vi "ncs_v4.vi"() -> ()   [LabVIEW 2016]
uses:
  <instrlib>/niUSRP/niUSRP Timestamp.ctl
  <vilib>/Analysis/3filter.llb/Filter Passband Type.ctl
  <instrlib>/niUSRP/niUSRP Write Tx Data (2D CDB).vi
  <instrlib>/niUSRP/niUSRP Fetch Rx Data (2D CDB).vi
  <vilib>/Analysis/baseanly.llb/IIR Cascade Filter (DBL).vi
  <vilib>/Analysis/NI_AALBase.lvlib
panel:
  in  "File Name":string="freq2G_1e"
  in  "Path":path=path "D:/Research/SummerFall17Spring18/CnC/NCS/Respiratory/Hexoskin/Data/3"
  out "NCS heartbeat":dbl[](graph)
  in  "Order":dbl=20.0 format="%#_13g"
  in  "High-Cutoff":dbl=8.0 format="%#_13g"
  in  "Low-Cutoff":dbl=0.5 format="%#_13g"
  out "size(s)":i32
  out "Coerced Rx IQ Rate":dbl
  in  "Sampling Rate":i32=500
  out "Gain":dbl=-15.0
  out "Bandwidth":dbl=56000000.0
  out "Coerced Carrier Freq":dbl=2000000000.0 format="%#.17g"
  out "Coerced Tx IQ rate":dbl=1000000.0
  out "error IO":errorcluster={"status"=FALSE, "code"=-1074118647, "source"=""}
  in  "Rx #Samples":i32=20000
  in  "Tab Control 2":enum32{"NI-294x/295x", "NI-2900/2901"}(tab)=enum."NI-2900/2901"
  in  "Rx carrier frequency [Hz]":dbl=2000000000.0 format="%#_6p"
  in  "Tx carrier frequency [Hz]":dbl=1000000000.0 format="%#_6p"
  in  "Start Trigger Time":T1={"whole seconds"=1, "fractional seconds"=0.0}
  in  "Tab Control":T2(tab)
  out "NCS tag Amp":dbl[](graph)=[0.011967714738528729, 0.012021355192189592, 0.012015275039596582, 0.011969166030167903, 0.011958890166168242, 0.012007893820858737, 0.012022893722444085, 0.011978222225113794, 0.011969989939463181, 0.012003099640895068]
  out "NCS tag Phase":dbl[](graph)=[0.011967714738528729, 0.012021355192189592, 0.012015275039596582, 0.011969166030167903, 0.011958890166168242, 0.012007893820858737, 0.012022893722444085, 0.011978222225113794, 0.011969989939463181, 0.012003099640895068]
  out "Tag Amp":dbl[](graph)
  out "Tag Phase":dbl[](graph)
  out "Tx Waveform Graph":waveform(dbl)[](graph)
  in  "Stop":bool
  in  "Tone Amplitude":dbl=0.707 step=0.05 format="%#.6g"
  in  "Tone Frequency":dbl=5000.0 format="%#_6p"
  in  "Tx Waveform Size":dbl=2000.0
  in  "Device Name":refnum<k15>="MyB210"
  in  "Tx Gain":dbl=28.0 format="%#_6f"
  in  "Tx IQ Rate":dbl=1000000.0 format="%#_6p"
  in  "Rx Gain":dbl=32.0 format="%#_6f"
  in  "Rx IQ Rate":dbl=500000.0 format="%#_6p"
  # "Note that on the NI-2900 and NI-2901, both Rx channels share an LO and both Tx channels share an LO. However, on the NI-294x/295x devices, Rx and Tx of channel 0 share an LO and Rx and Tx of channel 1 share an LO."
  # "Rx Settings"
  # "Tx Settings"
  # "Channel 0"
  # "Heartbeat Filter"
  # "This Tx graph should always have end and start tied up since this is being sent in a loop continuously. Otherwise phase jumps will be noticed."
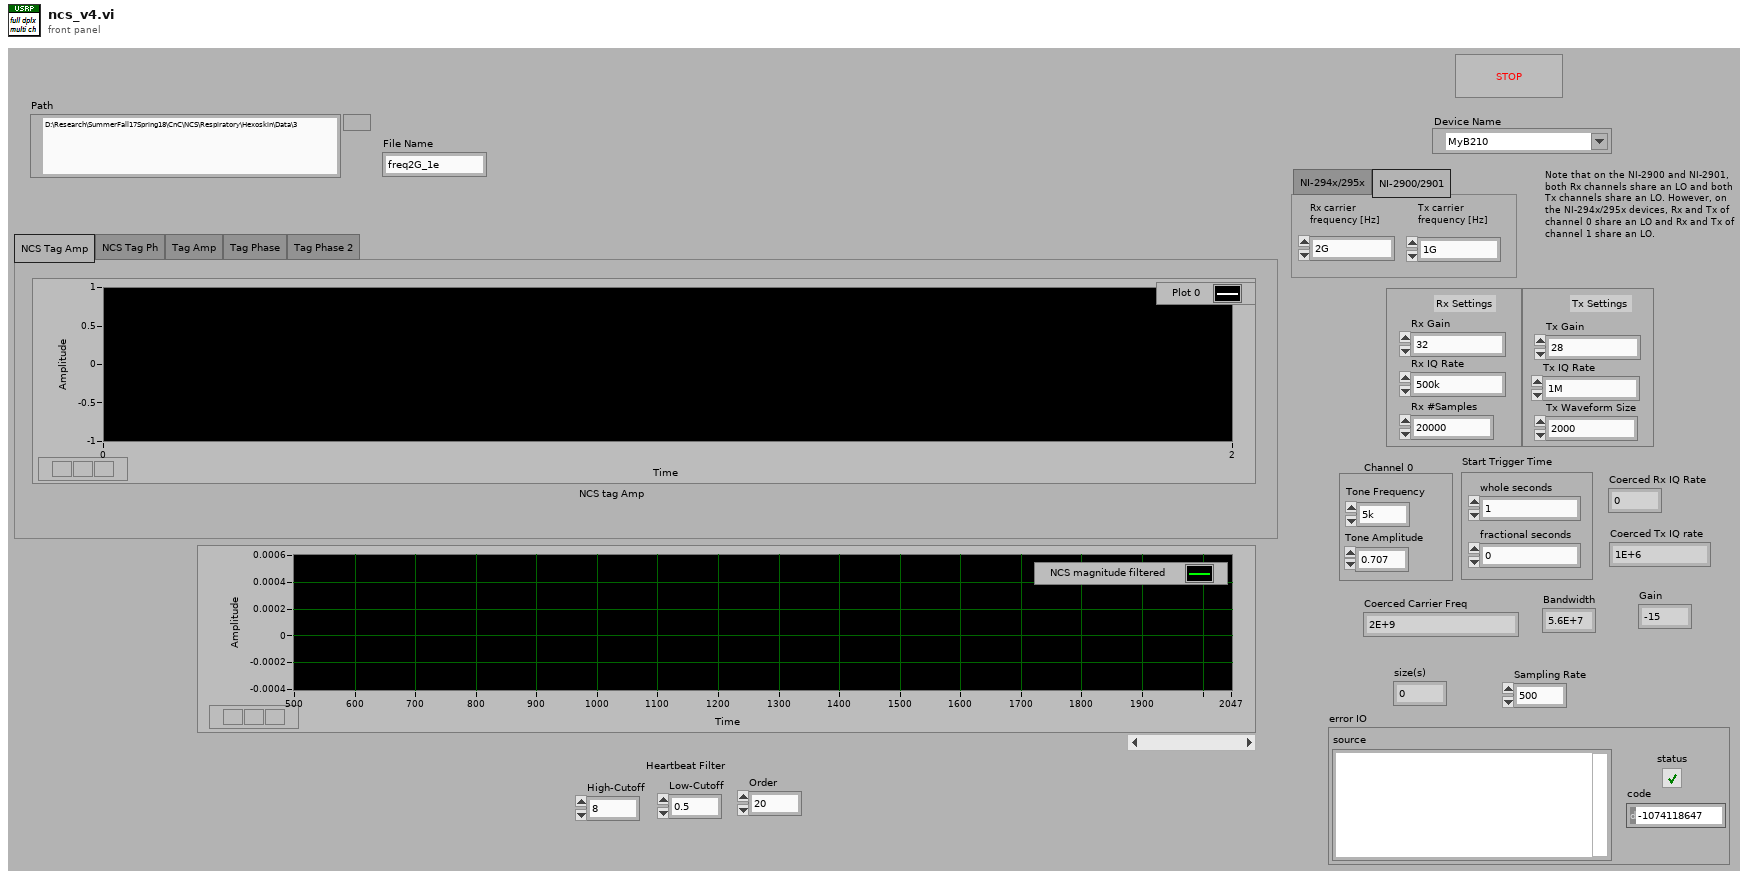
[diagram p1: front panel]
types:
  T1 = typedef "niUSRP Timestamp.ctl" = cluster{"whole seconds":u64, "fractional seconds":dbl}
  T2 = enum32{"NCS Tag Amp", "NCS Tag Ph", "Tag Amp", "Tag Phase", "Tag Phase 2"}
  T3 = typedef "NI_AALBase.lvlib/Filter Passband Type.ctl" = enum32{"Lowpass", "Highpass", "Bandpass", "Bandstop"}
  T4 = cluster{"filter structure":enum32{"IIR 2nd Order", "IIR 4th Order"}, "Reverse Coefficients":dbl[], "Forward Coefficients":dbl[]}
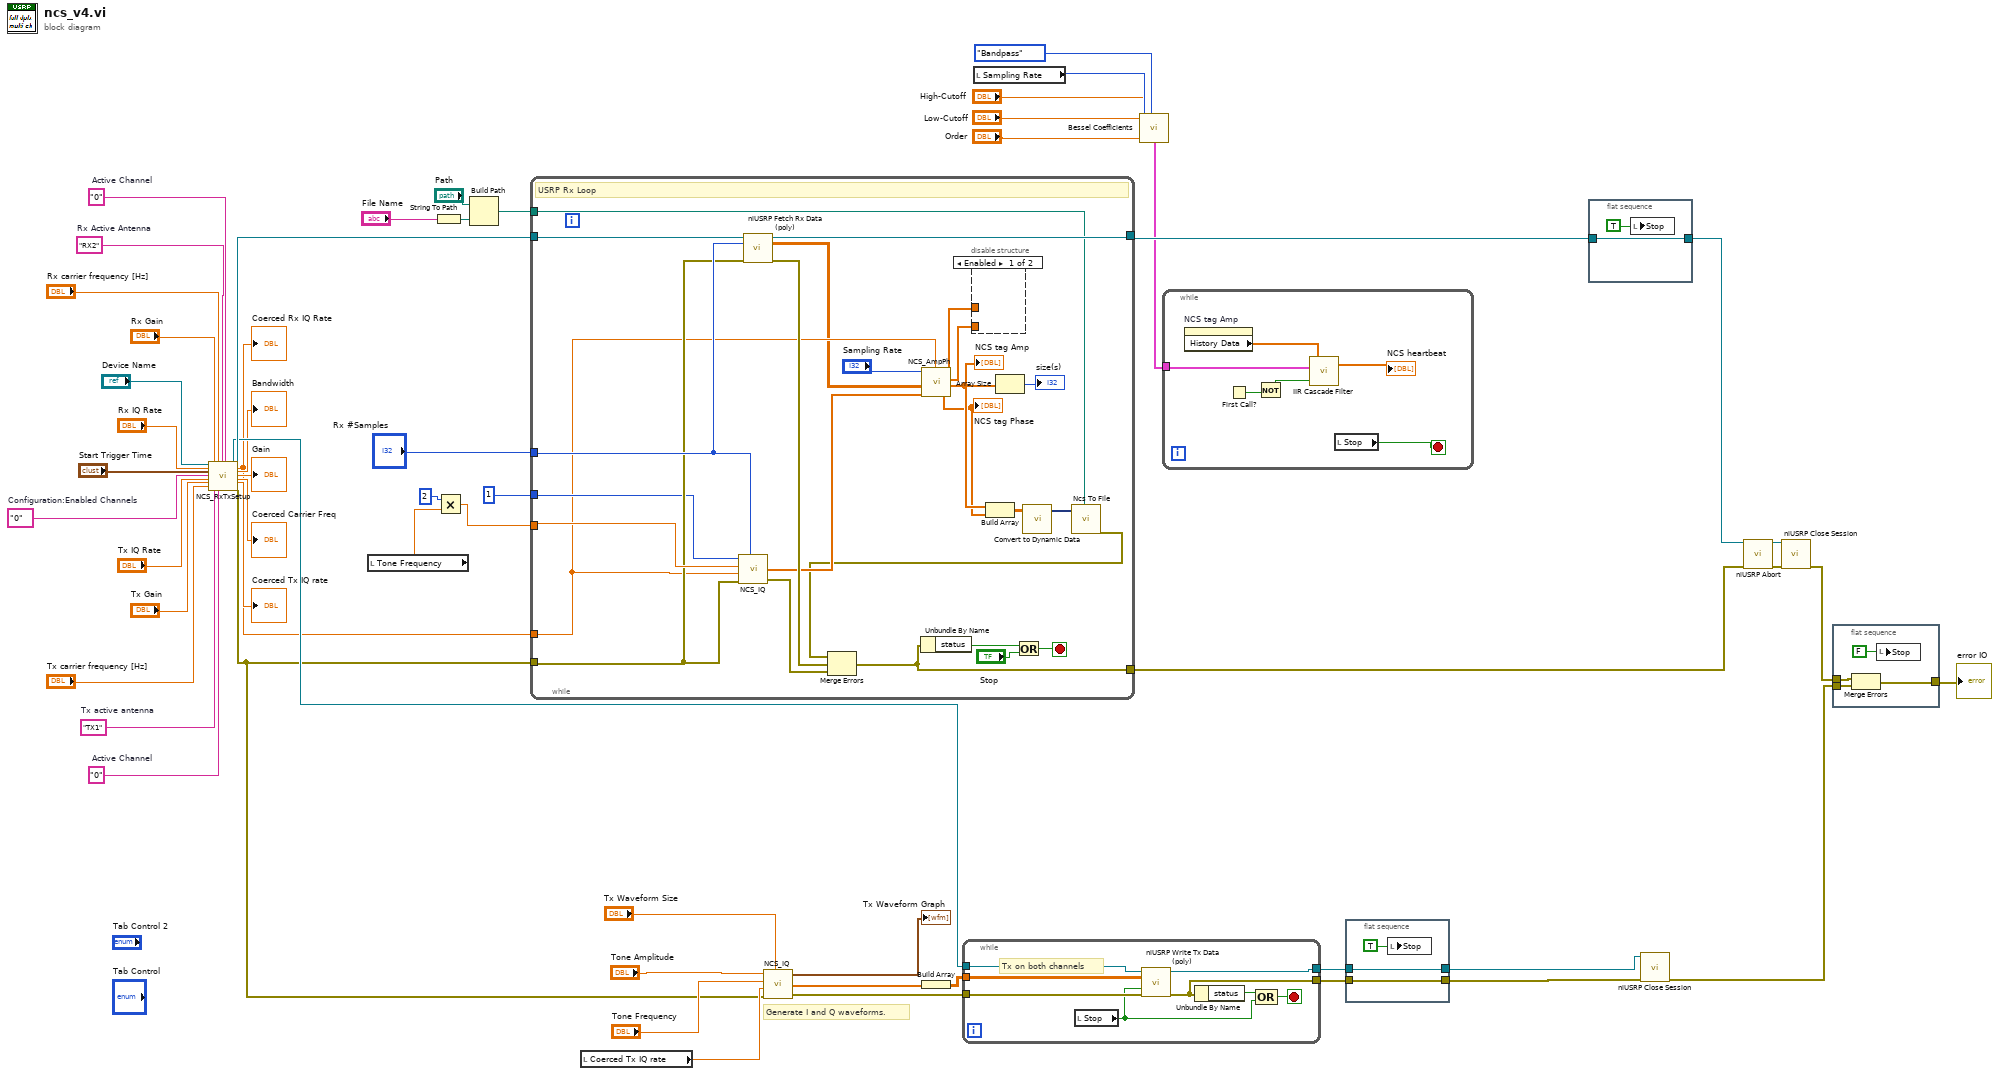
[diagram p0: block diagram]
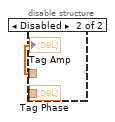
[diagram p2: hidden frame]
diagram:
  w12 = "0"  # Active Channel
  w13 = "0"  # Active Channel
  w48 = "RX2"  # Rx Active Antenna
  w44 = "TX1"  # Tx active antenna
  w30 = "0"  # Configuration:Enabled Channels
  # "Generate I and Q waveforms."
  n1 = call "NCS_RxTxSetup.vi"("IVI Refnum in"="Device Name", "Rx IQ Rate"="Rx IQ Rate", "Start Trigger Time"="Start Trigger Time", "Configuration:Enabled Channels"=w30, "Tx IQ Rate"="Tx IQ Rate", "Tx Gain"="Tx Gain", "Tx carrier frequency [Hz]"="Tx carrier frequency [Hz]", "Rx Gain"="Rx Gain", "Tx active antenna"=w44, "Rx carrier frequency [Hz]"="Rx carrier frequency [Hz]", "Active Channel"=w12, "Rx Active Antenna"=w48, "Active Channel 2"=w13) -> ("session handle out"=w55:refnum<k15>, "IVI Refnum out"=w56:refnum<k15>, "Coerced Rx IQ Rate"=w11:dbl, "Bandwidth"=→"Bandwidth":dbl, "Gain"=→"Gain":dbl, "Carrier Frequency"=→"Coerced Carrier Freq":dbl, "IQ Rate 2"=→"Coerced Tx IQ rate":dbl, "error out"=w23:errorcluster)  [unwired: 7 in]
  "Coerced Rx IQ Rate" <- w11
  n2 = local read "Tone Frequency"() -> (w29:dbl)
  n3 = String To Path(string="File Name") -> (path=w4:path)
  n4 = Multiply(x=2, y=w29) -> (x*y=w28:dbl)
  n5 = Build Path(base path="Path", name or relative path=w4) -> (appended path=w1:path)
  n6 = while {
    tunnel: w56 -> [w81]
    tunnel: w23 -> [w73]
    tunnel: [w80] -> w40
    tunnel: "Rx #Samples" -> [w75]
    tunnel: w11 -> [w69]
    tunnel: [w70] -> w32
    tunnel: w28 -> [w74]
    tunnel: 1 -> [w71]
    tunnel: w1 -> [w57]
    stop <- w76 stop-if-true
    # "USRP Rx Loop"
    n7 = call "NCS_IQ.vi"("Tone Amplitude"=w71, "Waveform Size"=w75, "Tone Frequency"=w74, "Coerced IQ rate"=w69, "error in (no error)"=w73) -> ("IQ waveform array"=w67:cdb[], "error out"=w72:errorcluster)  [unwired: 1 in, 1 out]
    n8 = call-poly <instrlib>:"niUSRP Fetch Rx Data (poly).vi"("session handle"=w81, "number of samples"=w75, "error in (no error)"=w73) -> ("session handle out"=w80:refnum<k15>, "data"=w68:cdb[][], "error out"=w77:errorcluster)  [unwired: 9 in, 1 out]
    n9 = call "NCS_AmpPh.vi"("IQ"=w67, "data"=w68, "Sampling Rate"="Sampling Rate", "Coerced Rx IQ Rate"=w69) -> ("Phase DownSampled"=w60:dbl[], "Amp DownSampled"=w61:dbl[], "Unfiltered Phase"=w66:dbl[], "Unfiltered Amplitude"=w64:dbl[])  [unwired: 4 in]
    "NCS tag Amp" <- w61
    "NCS tag Phase" <- w60
    n10 = disable-structure shown="Enabled" {
      disable-tunnel: w64 -> [_ w83]
      disable-tunnel: w66 -> [_ w82]
      frame Enabled {
      }
      frame Disabled {
        "Tag Amp" <- w83
        "Tag Phase" <- w82
      }
    }
    n11 = Build Array(w61, w60) -> (w62:dbl[][])
    n12 = Array Size(array=w61) -> (size(s)=→"size(s)":i32)
    n13 = call "Convert to Dynamic Data"("2D Array"=w62) -> ("Dynamic Data Type"=w59:dynamicdata)  [unwired: 3 in]
    n14 = call "Ncs To File"("Signals"=w59, "Filename"=w57) -> ("error out"=w58:errorcluster)  [unwired: 15 in, 2 out]
    n15 = Merge Errors(w58, w77, w72) -> (w70:errorcluster)
    n16 = Unbundle By Name(w70) -> ("status"=w79:bool)
    n17 = Or(x=w79, y="Stop") -> (x .or. y?=w76:bool)
  }
  n18 = local read "Coerced Tx IQ rate"() -> (w24:dbl)
  n19 = call "NCS_IQ.vi"("Tone Amplitude"="Tone Amplitude", "Waveform Size"="Tx Waveform Size", "Tone Frequency"="Tone Frequency", "Coerced IQ rate"=w24, "error in (no error)"=w23) -> ("IQ waveform"=→"Tx Waveform Graph":waveform(dbl)[], "IQ waveform array"=w21:cdb[], "error out"=w22:errorcluster)  [unwired: 1 in]
  n20 = Build Array(w21) -> (w52:cdb[][])
  n21 = while {
    tunnel: w55 -> [w91]
    tunnel: w22 -> [w90]
    tunnel: [w88] -> w43
    tunnel: [w86] -> w38
    tunnel: w52 -> [w84]
    stop <- w87 stop-if-true
    # "Tx on both channels"
    n22 = local read "Stop"() -> (w85:bool)
    n23 = call-poly <instrlib>:"niUSRP Write Tx Data (poly).vi"("session handle"=w91, "data"=w84, "end of data?"=w85, "error in (no error)"=w90) -> ("session handle out"=w86:refnum<k15>, "error out"=w88:errorcluster)  [unwired: 10 in]
    n24 = Unbundle By Name(w88) -> ("status"=w89:bool)
    n25 = Compound Arithmetic op=OR(w89, w85) -> (w87:bool)
  }
  n26 = local read "Sampling Rate"() -> (w9:i32)
  n27 = call <vilib>:"Bessel Coefficients.vi"("order"="Order", "filter type"=Filter_Passband_Type."Bandpass", "low cutoff freq: fl"="Low-Cutoff", "high cutoff freq: fh"="High-Cutoff", "sampling freq: fs"=w9) -> ("IIR Filter Cluster"=w5:T4)  [unwired: 5 in, 1 out]
  n28 = while {
    tunnel: w5 -> [w94]
    stop <- w96 stop-if-true
    n29 = property on="NCS tag Amp" class="WaveformChart (strict)"() -> ("History Data"=w95:dbl[])  [unwired: 2 in, 2 out]
    n30 = First Call?() -> (First Call?: T/F=w97:bool)
    n31 = Not(x=w97) -> (.not. x?=w93:bool)
    n32 = call-poly <vilib>:"IIR Cascade Filter.vi"("init/cont (init:F)"=w93, "IIR Filter Cluster"=w94, "X"=w95) -> ("Filtered X"=→"NCS heartbeat":dbl[])  [unwired: 1 out]
    n33 = local read "Stop"() -> (w96:bool)
  }
  n34 = flat-sequence {
    tunnel: [w99] -> w42
    tunnel: w43 -> [w99]
    tunnel: [w98] -> w39
    tunnel: w38 -> [w98]
    frame #0 {
      n35 = local write "Stop"(TRUE ("STOP")) -> ()
    }
  }
  n36 = flat-sequence {
    tunnel: [w101] -> w41
    tunnel: w40 -> [w101]
    frame #0 {
      n37 = local write "Stop"(TRUE ("STOP")) -> ()
    }
  }
  n38 = call <instrlib>:"niUSRP Close Session.vi"("session handle"=w39, "error in (no error)"=w42) -> ("error out"=w37:errorcluster)  [unwired: 13 in]
  n39 = call <instrlib>:"niUSRP Abort.vi"("session handle"=w41, "error in (no error)"=w32) -> ("session handle out"=w54:refnum<k15>, "error out"=w53:errorcluster)  [unwired: 12 in]
  n40 = call <instrlib>:"niUSRP Close Session.vi"("session handle"=w54, "error in (no error)"=w53) -> ("error out"=w34:errorcluster)  [unwired: 13 in]
  n41 = flat-sequence {
    tunnel: w37 -> [w105]
    tunnel: [w104] -> w35
    tunnel: w34 -> [w103]
    frame #0 {
      n42 = Merge Errors(w103, w105) -> (w104:errorcluster)
      n43 = local write "Stop"(FALSE ("STOP")) -> ()
    }
  }
  "error IO" <- w35
